vi "Refresh2DGraph.vi"(6 "Data":dbl[](array[numeric]), 8 "error in (no error)":errorcluster caption="entrée d'erreur (pas d'erreur)", 9 "CurveIndex":i32, 10 "PointIndex":i32, 11 "Interface en entrée":refnum<class "Interface.lvclass"> caption="DNL_LabVIEW Object in") -> (0 "error out":errorcluster caption="sortie d'erreur", 3 "Interface en sortie":refnum<class "Interface.lvclass"> caption="DNL_LabVIEW Object out")   [LabVIEW 2019, in "Interface.lvclass"]
uses:
  Interface.lvclass
  Interface.lvclass/Interface.ctl
  2DGraphQData.ctl
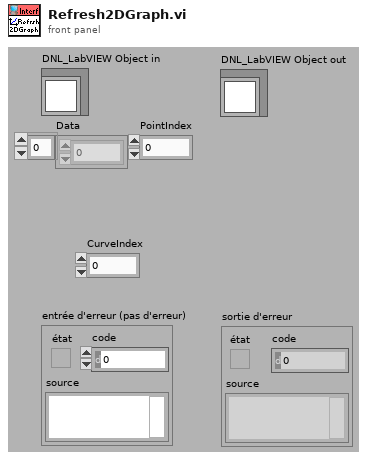
[diagram p1: front panel]
types:
  T1 = typedef "2DGraphQData.ctl" = cluster{"X Ind(Line)":i32, "Y Ind(Col)":i32, "Data":dbl}
  T2 = typedef "2DGraphSetup.ctl" = cluster{"ZDataIndex":i32, "XParIndex":i32, "YParIndex":i32, "FillLineFirst":bool}
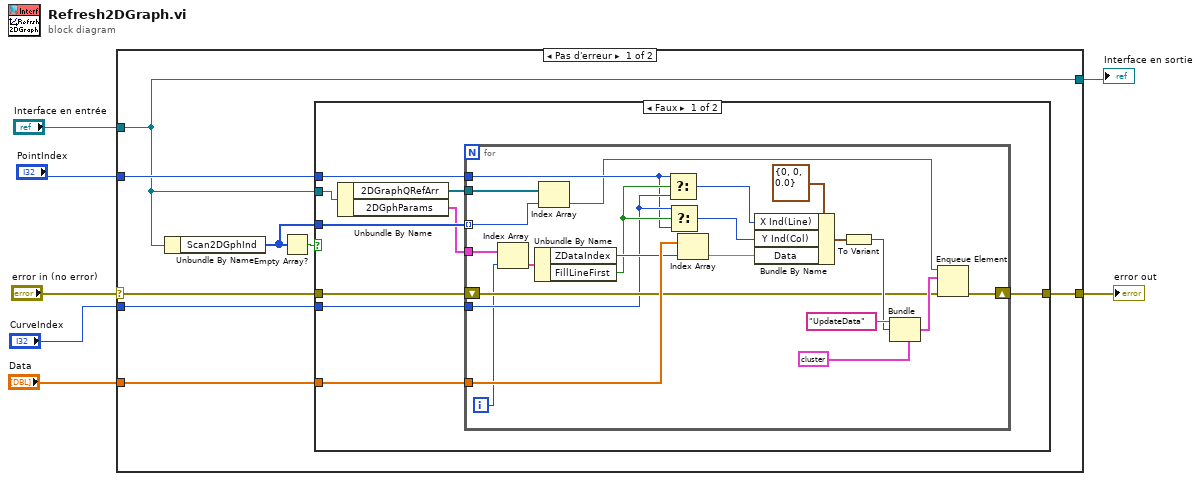
[diagram p0: block diagram]
diagram:
  n1 = case shown="Pas d'erreur" "error in (no error)" {
    selector: "error in (no error)" -> [w15 w49]
    tunnel: [w14 w49] -> w6
    tunnel: [w9 w48] -> w4
    tunnel: "Interface en entrée" -> [w9 w48]
    tunnel: "CurveIndex" -> [w12 _]
    tunnel: "Data" -> [w11 _]
    tunnel: "PointIndex" -> [w10 _]
    frame No Error {
      n2 = Unbundle By Name(w9) -> ("Scan2DGphInd"=w8:i32[])
      n3 = Empty Array?(array=w8) -> (empty?=w13:bool)
      n4 = case shown="Faux" w13 {
        tunnel: w9 -> [w24 _]
        tunnel: w15 -> [w23 w47]
        tunnel: [w20 w47] -> w14
        tunnel: w12 -> [w22 _]
        tunnel: w11 -> [w19 _]
        tunnel: w10 -> [w18 _]
        tunnel: w8 -> [w17 _]
        frame False {
          n5 = Unbundle By Name(w24) -> ("2DGraphQRefArr"=w21:refnum<queue>[], "2DGphParams"=w16:T2[])
          n6 = for {
            tunnel: w17 -> [w40] mode=indexing
            shift-right: [w41] -> w20
            shift-left: w23 -> [w30]
            tunnel: w16 -> [w46]
            tunnel: w22 -> [w29]
            tunnel: w21 -> [w39]
            tunnel: w19 -> [w38]
            tunnel: w18 -> [w28]
            i -> [w25]
            n7 = Index Array(array=w46, index=w25) -> (element=w45:T2)
            n8 = Unbundle By Name(w45) -> ("ZDataIndex"=w37:i32, "FillLineFirst"=w32:bool)
            n9 = Index Array(array=w39, index=w40) -> (element=w26:refnum<queue>)
            n10 = Select(t=w28, s=w32, f=w29) -> (s? t:f=w31:i32)
            n11 = Select(t=w29, s=w32, f=w28) -> (s? t:f=w27:i32)
            n12 = Index Array(array=w38, index=w37) -> (element=w33:dbl)
            n13 = Bundle By Name(cluster=T1 {"X Ind(Line)"=0, "Y Ind(Col)"=0, "Data"=0.0} ("2DGphQData"), "X Ind(Line)"=w31, "Y Ind(Col)"=w27, "Data"=w33) -> (w35:T1)
            n14 = To Variant(anything=w35) -> (Variant=w34:variant)
            n15 = Bundle(cluster=cluster{"Message":string, "Data":variant, i32} {"Message"="", "Data"=variant, 0} ("élément"), "Message"="UpdateData", "Data"=w34) -> (w43:cluster{"Message":string, "Data":variant, i32})  [unwired: 1 in]
            n16 = Enqueue Element(queue=w26, element=w43, error in (no error)=w30) -> (error out=w41:errorcluster)  [unwired: 1 in, 2 out]
          }
        }
        frame True {
        }
      }
    }
    frame Error {
    }
  }
  "error out" <- w6
  "Interface en sortie" <- w4
